vi "Day3.vi"(11 "Input":string) -> (3 "Result":i64)   [LabVIEW 2024]
uses:
  <vilib>/regexp/Match Regular Expression.xnode
panel:
  out "Array":string[](array[string])
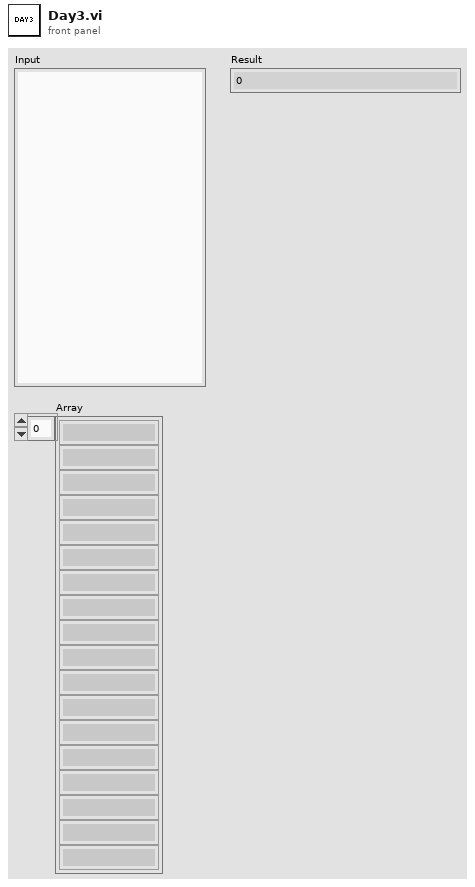
[diagram p1: front panel]
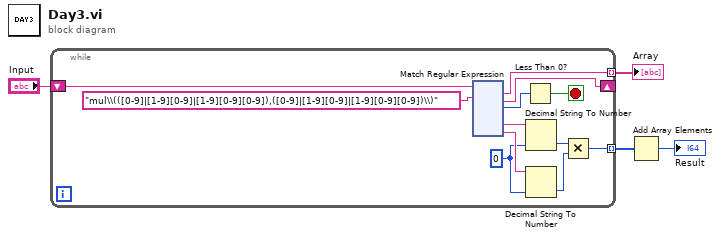
[diagram p0: block diagram]
diagram:
  n1 = while {
    shift-right: [w14] -> _
    shift-left: "Input" -> [w16]
    tunnel: [w9] -> w4 mode=indexing
    tunnel: [w7] -> w2 mode=indexing
    stop <- w5 stop-if-true
    w8 = i64 0 ("default (0 I32)")
    n2 = xnode "Match Regular Expression"("input string"=w16, "regular expression"="mul\\(([0-9]|[1-9][0-9]|[1-9][0-9][0-9]),([0-9]|[1-9][0-9]|[1-9][0-9][0-9])\\)") -> ("whole match"=w7:string, "after match"=w14:string, "offset past match"=w6:i32, "submatch 1"=w13:string, "submatch 2"=w12:string)  [unwired: 4 in, 2 out]
    n3 = Less Than 0?(x=w6) -> (x < 0?=w5:bool)
    n4 = Decimal String To Number(string=w13, default (0L)=w8) -> (number=w11:i64)  [unwired: 1 in, 1 out]
    n5 = Decimal String To Number(string=w12, default (0L)=w8) -> (number=w10:i64)  [unwired: 1 in, 1 out]
    n6 = Multiply(x=w11, y=w10) -> (x*y=w9:i64)
  }
  "Array" <- w2
  n7 = Add Array Elements(numeric array=w4) -> (sum=→"Result":i64)
